vi "cadena de luces.vi"() -> ()   [LabVIEW 2019]
panel:
  out "Numeric":dbl
  in  "Array":bool[](array[boolean])
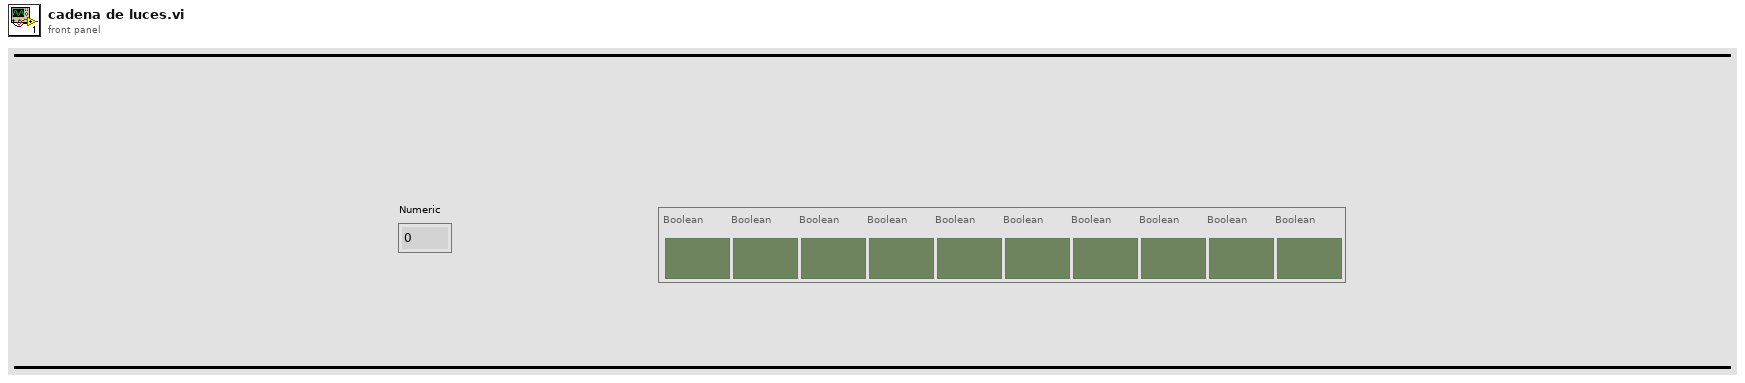
[diagram p1: front panel]
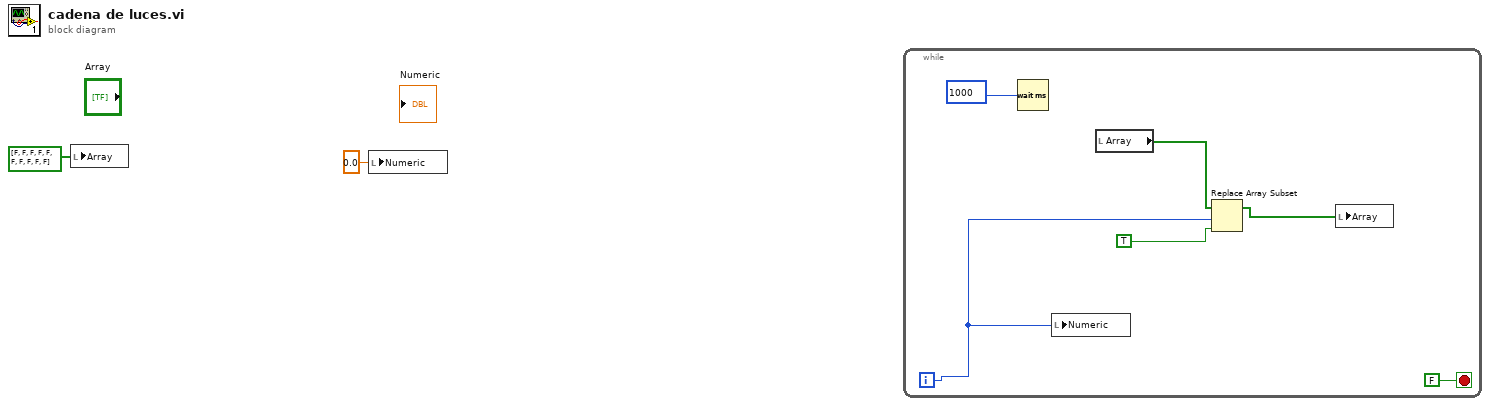
[diagram p0: block diagram]
diagram:
  n1 = local write "Array"(bool[] [FALSE, FALSE, FALSE, FALSE, FALSE, FALSE, FALSE, FALSE, FALSE, FALSE] ("Array")) -> ()
  n2 = local write "Numeric"(0.0 ("Numeric")) -> ()
  n3 = while {
    i -> [w3]
    stop <- FALSE stop-if-true
    n4 = Wait (ms)(milliseconds to wait=u32 1000 ("millisecond timer value")) -> ()  [unwired: 1 out]
    n5 = local write "Numeric"(w3) -> ()
    n6 = local read "Array"() -> (w4:bool[])
    n7 = Replace Array Subset(array=w4, new element=TRUE, index=w3) -> (w5:bool[])
    n8 = local write "Array"(w5) -> ()
  }
